vi "Folder_SPCImporter_CWB_FDA.vi"(1 "Select folder with  .spc files to convert to one .csv file that contains the Raman data and one .csv file that contains to instrument information.":path=path "" caption="start path") -> (0 "SPECTRA":cluster{i32[], i32[]}(graph))   [LabVIEW 2015]
uses:
  <vilib>/Utility/file.llb/Write To Spreadsheet File (string).vi
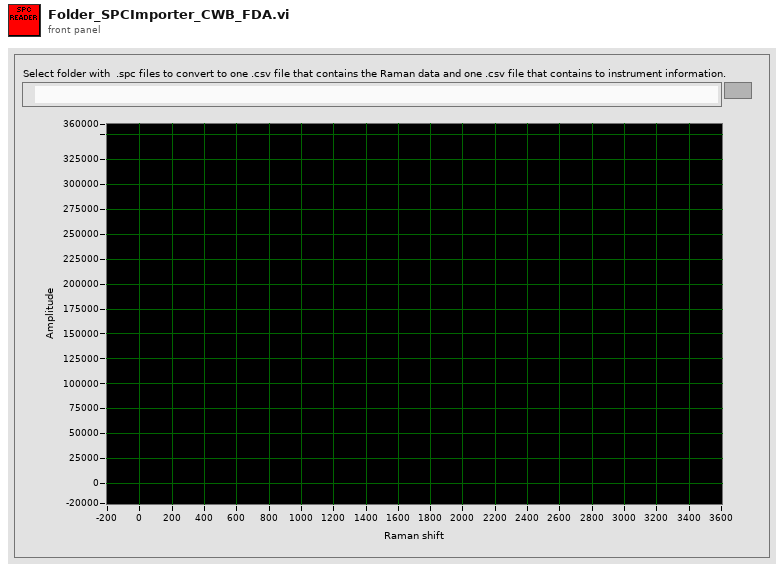
[diagram p1: front panel]
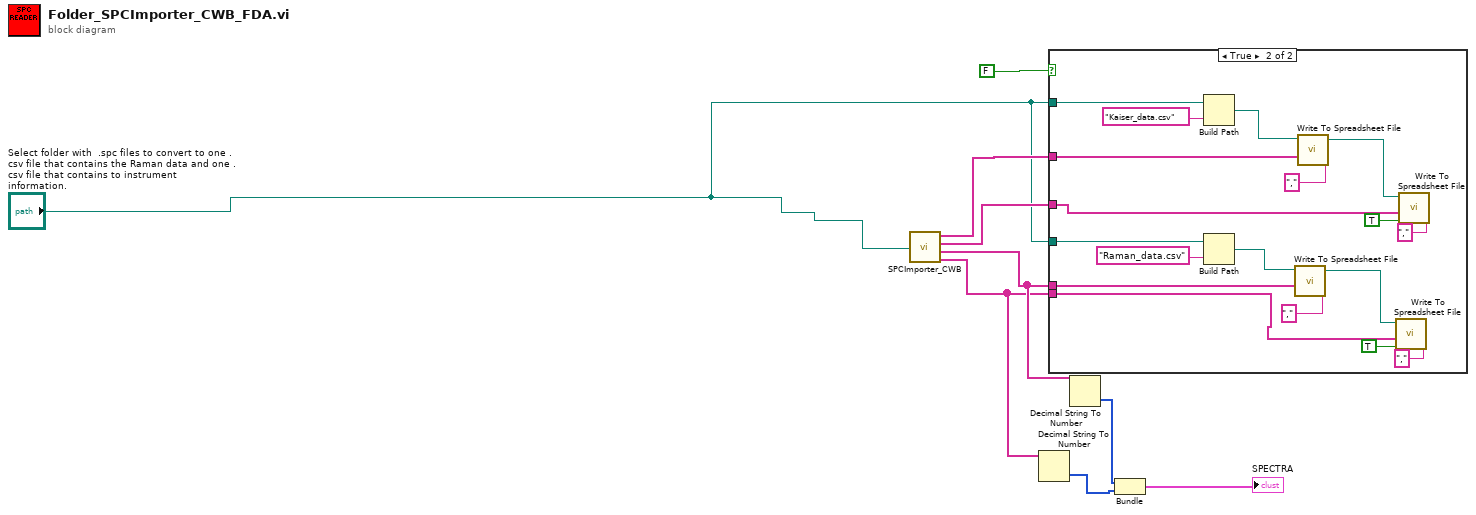
[diagram p0: block diagram]
diagram:
  n1 = call "SPCImporter_CWB.vi"("start path"="Select folder with  .spc files to convert to one .csv file that contains the Raman data and one .csv file that contains to instrument information.") -> ("Kaiser labels"=w9:string[], "Kaiser data"=w8:string[], "Raman labels"=w7:string[], "Raman data"=w6:string[])
  n2 = Decimal String To Number(string=w6) -> (number=w1:i32[])  [unwired: 2 in, 1 out]
  n3 = case shown="True" FALSE {
    tunnel: w9 -> [_ w16]
    tunnel: "Select folder with  .spc files to convert to one .csv file that contains the Raman data and one .csv file that contains to instrument information." -> [_ w15]
    tunnel: w8 -> [_ w11]
    tunnel: w7 -> [_ w13]
    tunnel: w6 -> [_ w10]
    tunnel: "Select folder with  .spc files to convert to one .csv file that contains the Raman data and one .csv file that contains to instrument information." -> [_ w12]
    frame False {
    }
    frame True {
      n4 = Build Path(base path=w12, name or relative path="Kaiser_data.csv") -> (appended path=w17:path)
      n5 = Build Path(base path=w15, name or relative path="Raman_data.csv") -> (appended path=w22:path)
      n6 = call-poly <vilib>:"Write To Spreadsheet File.vi"("delimiter (\\t)"="," ("delimiter (\\t)"), "1D data"=w13, "file path (dialog if empty)"=w22) -> ("new file path (Not A Path if cancelled)"=w23:path)  [unwired: 5 in]
      n7 = call-poly <vilib>:"Write To Spreadsheet File.vi"("delimiter (\\t)"="," ("delimiter (\\t)"), "1D data"=w16, "file path (dialog if empty)"=w17) -> ("new file path (Not A Path if cancelled)"=w18:path)  [unwired: 5 in]
      n8 = call-poly <vilib>:"Write To Spreadsheet File.vi"("delimiter (\\t)"="," ("delimiter (\\t)"), "append to file? (new file:F)"=TRUE, "1D data"=w10, "file path (dialog if empty)"=w23) -> ()  [unwired: 4 in, 1 out]
      n9 = call-poly <vilib>:"Write To Spreadsheet File.vi"("delimiter (\\t)"="," ("delimiter (\\t)"), "append to file? (new file:F)"=TRUE, "1D data"=w11, "file path (dialog if empty)"=w18) -> ()  [unwired: 4 in, 1 out]
    }
  }
  n10 = Decimal String To Number(string=w7) -> (number=w5:i32[])  [unwired: 2 in, 1 out]
  n11 = Bundle(w5, w1) -> (→"SPECTRA":cluster{i32[], i32[]})  [unwired: 1 in]
